vi "test Update Series View 1.vi"(11 "Test Case In":refnum<class "test Update Series View.lvclass">) -> (0 "error out":errorcluster, 3 "Test Case Out":refnum<class "test Update Series View.lvclass">)   [LabVIEW 2023, in "test Update Series View.lvclass"]
uses:
  test Update Series View.lvclass
  C:/Program Files/National Instruments/LabVIEW 2023/vi.lib/Astemes/LUnit/Test Case.lvclass
  source/Series Graph/Graph with Series View.lvclass
  D:/git/Lock-In-Thermography-Graphs/source/Base Graph/Base Graph.lvclass
  source/Base Graph/Base Graph.lvclass/Base Graph.ctl
  source/Series Graph/Graph with Series View.lvclass/Graph with Series View.ctl
  <vilib>/Astemes/LUnit/Test Case.lvclass/Test Case.ctl
  source/Series Graph/Get 1D Array Image Index and Length.vi
  source/Base Graph/Get Size.vi
  <vilib>/Astemes/LUnit/Append Fail Result.vi
  <vilib>/Astemes/LUnit/Append Pass Result.vi
  <vilib>/Astemes/LUnit/Run In UI.vi
  <vilib>/Utility/error.llb/Clear Errors.vi
  test Update Series View.lvclass/test Update Series View.ctl
  <vilib>/Analysis/NI_AALBase.lvlib
  source/Base Graph/Base Graph.lvclass
  <vilib>/Astemes/LUnit/Test Case.lvclass
panel:
  out "Z - Time Signal":dbl[](graph)
  out "Intensity Width Graph":cluster{"Array":dbl[], "Array":dbl[]}(graph)
  out "Signal Map":u16[][](graph)
  out "Intensity Height Graph":cluster{"Array":dbl[], "Array":dbl[]}(graph)
  in  "Image #":u16
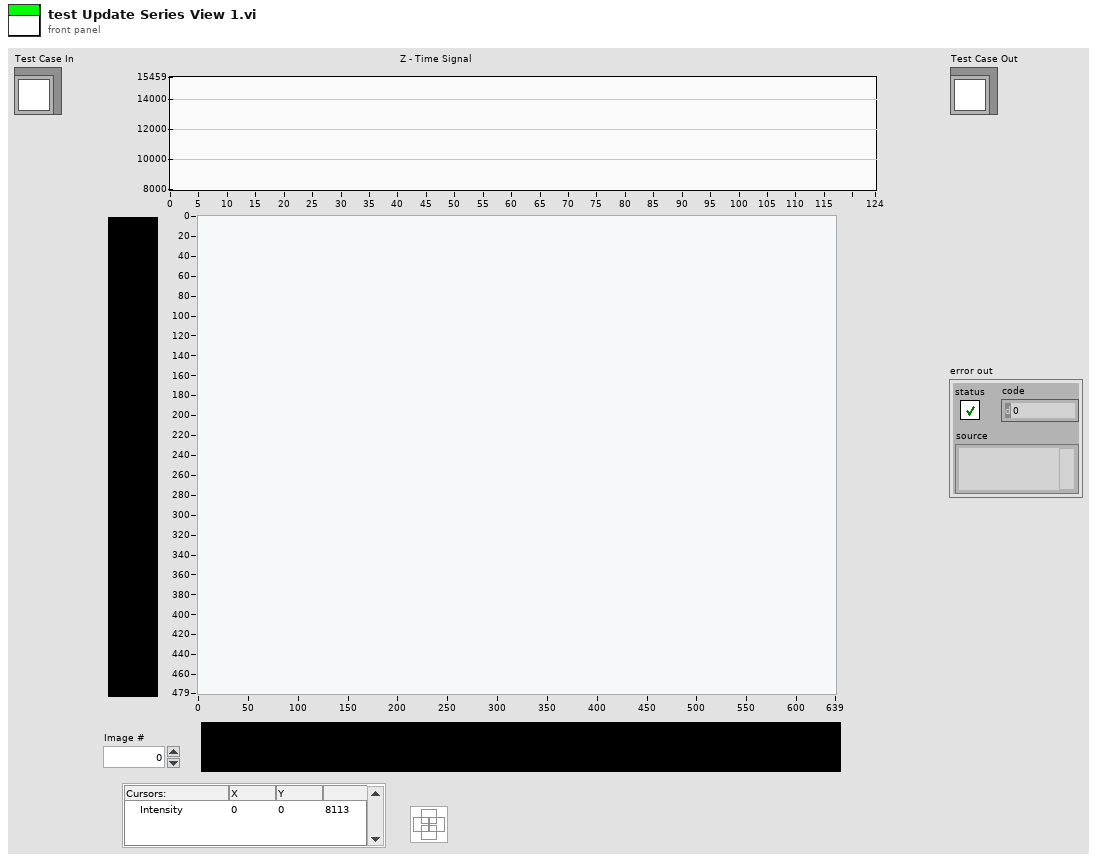
[diagram p1: front panel]
types:
  T1 = cluster{"Z-Graph":refnum<vi>, "IntGraph":refnum<vi>, "Y-Graph":refnum<vi>, "X-Graph":refnum<vi>}
  T2 = typedef "LVPointDoubleTypeDef.ctl" = cluster{"X":dbl, "Y":dbl}
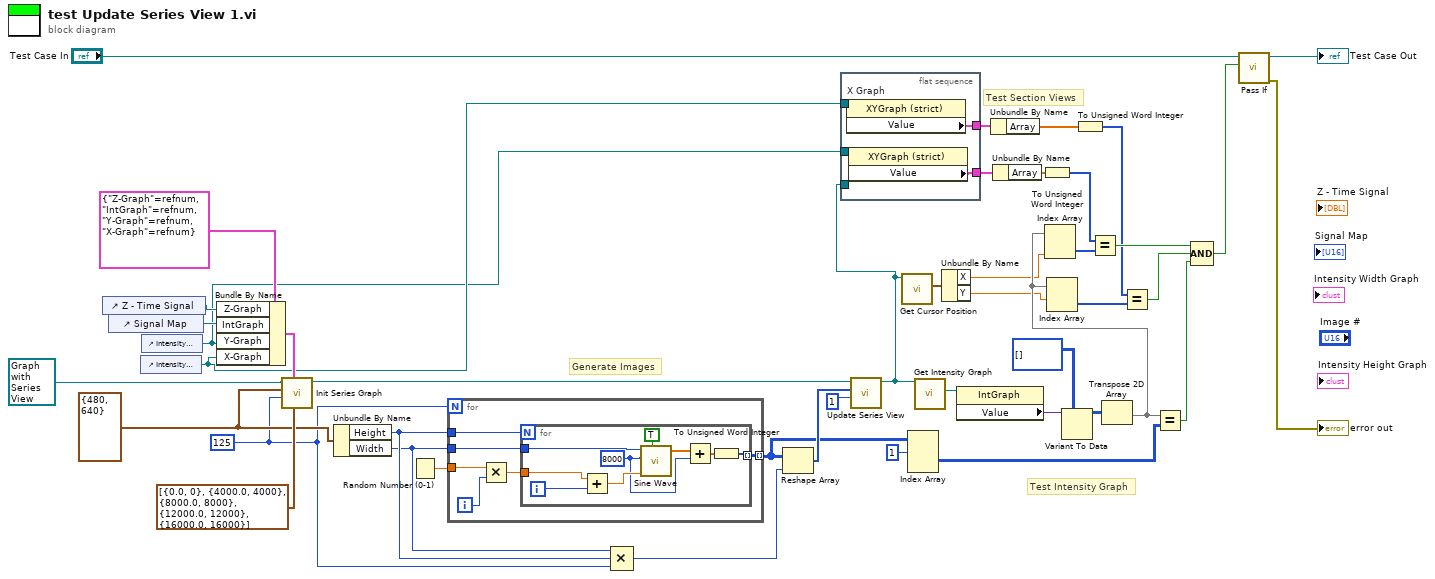
[diagram p0: block diagram]
diagram:
  w32 = u32 125 ("Shots")
  w35 = cluster{"Height":u32, "Width":u32} {"Height"=480, "Width"=640} ("Images Size")
  # "Generate Images"
  # "Test Intensity Graph"
  # "Test Section Views"
  n1 = control-ref of="Z - Time Signal"() -> (w37:refnum<vi>)
  n2 = control-ref of="Signal Map"() -> (w36:refnum<vi>)
  n3 = control-ref of="Intensity Width Graph"() -> (w13:refnum<vi>)
  n4 = control-ref of="Intensity Height Graph"() -> (w12:refnum<vi>)
  n5 = Bundle By Name(cluster=T1 {"Z-Graph"=refnum, "IntGraph"=refnum, "Y-Graph"=refnum, "X-Graph"=refnum} ("Graphs"), "Z-Graph"=w37, "IntGraph"=w36, "Y-Graph"=w12, "X-Graph"=w13) -> (w40:T1)
  n6 = call "Init Series Graph.vi"("Z Scale.Marker Values[]"=cluster{"Numeric":dbl, "Numeric":u32}[] [{"Numeric"=0.0, "Numeric"=0}, {"Numeric"=4000.0, "Numeric"=4000}, {"Numeric"=8000.0, "Numeric"=8000}, {"Numeric"=12000.0, "Numeric"=12000}, {"Numeric"=16000.0, "Numeric"=16000}], "Graphs"=w40, "Shots"=w32, "Image Size"=w35, "Series Graph in"=refnum<class "Graph with Series View.lvclass"> refnum) -> ("Series Graph out"=w14:refnum<class "Graph with Series View.lvclass">)  [unwired: 5 in, 1 out]
  n7 = Unbundle By Name(w35) -> ("Height"=w34:u32, "Width"=w33:u32)
  n8 = Random Number (0-1)() -> (number: 0 to 1=w22:dbl)
  n9 = for {
    N: w32 -> [_]
    tunnel: [w50] -> w26 mode=indexing
    tunnel: w33 -> [w49]
    tunnel: w34 -> [w48]
    tunnel: w22 -> [w46]
    i -> [w47]
    n10 = Multiply(x=w46, y=w47) -> (x*y=w45:dbl)
    n11 = for {
      N: w48 -> [_]
      tunnel: [w51] -> w50 mode=indexing
      tunnel: w49 -> [w55]
      tunnel: w45 -> [w53]
      i -> [w58]
      w54 = u16 8000 ("amplitude")
      n12 = Add(x=w53, y=w58) -> (x+y=w57:dbl)
      n13 = call <vilib>:"Sine Wave.vi"("samples"=w55, "amplitude"=w54, "phase in"=w57, "reset phase"=TRUE) -> ("sine wave"=w52:dbl[])  [unwired: 1 in, 2 out]
      n14 = Add(x=w52, y=w54) -> (x+y=w56:dbl[])
      n15 = To Unsigned Word Integer(number=w56) -> (unsigned 16bit integer=w51:u16[])
    }
  }
  n16 = Compound Arithmetic op=MULTIPLY(w33, w34, w32) -> (w31:u32)
  n17 = Reshape Array(w26, w31) -> (w30:u16[])
  n18 = flat-sequence {
    tunnel: w12 -> [w63]
    tunnel: w13 -> [w62]
    tunnel: [w61] -> w21
    tunnel: [w60] -> w20
    tunnel: w9 -> [_]
    frame #0 {
      n19 = property on="X Graph" class="XYGraph (strict)"(reference=w62) -> ("Value"=w61:cluster{"Array":dbl[], "Array":dbl[]})  [unwired: 1 in, 2 out]
      n20 = property class="XYGraph (strict)"(reference=w63) -> ("Value"=w60:cluster{"Array":dbl[], "Array":dbl[]})  [unwired: 1 in, 2 out]
    }
  }
  n21 = call "Update Series View.vi"("Image #"=u32 1, "Image Series"=w30, "Series Graph in"=w14) -> ("Series Graph out"=w9:refnum<class "Graph with Series View.lvclass">)  [unwired: 8 in]
  n22 = call "Get Cursor Position.vi"("Base Graph in"=w9) -> ("Cursor Position"=w19:T2)  [unwired: 9 in, 1 out]
  n23 = Index Array(array=w26, index (dim 0)=1 ("index (page)")) -> (element=w23:u16[][])  [unwired: 2 in]
  n24 = call "Get Intensity Graph.vi"("Base Graph in"=w9) -> ("Intensity Graph"=w11:refnum<vi>)  [unwired: 9 in, 1 out]
  n25 = Unbundle By Name(w19) -> ("X"=w4:dbl, "Y"=w3:dbl)
  n26 = property class="IntGraph"(reference=w11) -> ("Value"=w28:variant)  [unwired: 1 in, 2 out]
  n27 = Unbundle By Name(w21) -> ("Array"=w15:dbl[])
  n28 = Unbundle By Name(w20) -> ("Array"=w17:dbl[])
  n29 = To Unsigned Word Integer(number=w17) -> (unsigned 16bit integer=w1:u16[])
  n30 = Variant To Data(type=u16[][] [], Variant=w28) -> (data=w24:u16[][])  [unwired: 1 in, 1 out]
  n31 = To Unsigned Word Integer(number=w15) -> (unsigned 16bit integer=w2:u16[])
  n32 = Transpose 2D Array(2D array=w24) -> (transposed array=w10:u16[][])
  n33 = Index Array(array=w10, index (col)=w4) -> (element=w18:u16[])  [unwired: 1 in]
  n34 = Index Array(array=w10, index (row)=w3) -> (element=w16:u16[])  [unwired: 1 in]
  n35 = Equal?(x=w1, y=w18) -> (x = y?=w7:bool)
  n36 = Equal?(x=w2, y=w16) -> (x = y?=w6:bool)
  n37 = Equal?(x=w10, y=w23) -> (x = y?=w5:bool)
  n38 = Compound Arithmetic op=AND(w7, w6, w5) -> (w8:bool)
  n39 = call <vilib>:"Pass If.vi"("Pass?"=w8, "LUnit Test Case In"="Test Case In") -> ("error out"=→"error out":errorcluster, "LUnit Test Case Out"=→"Test Case Out":refnum<class "test Update Series View.lvclass">)  [unwired: 8 in]
